vi "Correct U16 Image Array.vi"(8 "Error In":errorcluster, 11 "Image Pixels (U16)":u16[][](array[numeric])) -> (0 "Error Out":errorcluster, 3 "Corrected Image Pixels (U16)":u16[][](array[numeric]))   [LabVIEW 2021, in "Image.lvlib"]
doc: "Subtract 32768 from a U16 array if that it its minimum, as is the case for image data read from TIFF files"
uses:
  Image/Image.lvlib
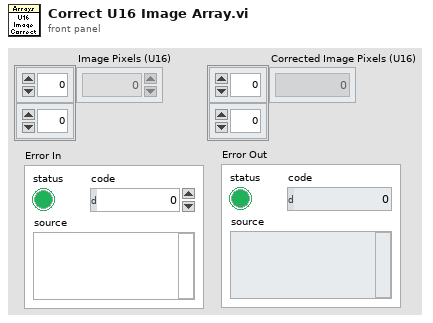
[diagram p1: front panel]
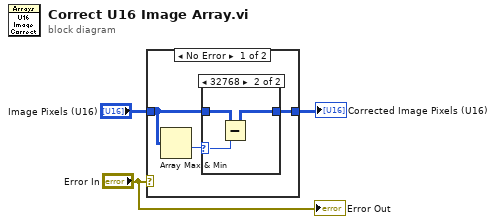
[diagram p0: block diagram]
diagram:
  n1 = case shown="No Error" "Error In" {
    tunnel: "Image Pixels (U16)" -> [w5 w11]
    tunnel: [w4 w11] -> w2
    frame No Error {
      n2 = Array Max & Min(array=w5) -> (min value=w6:u16)  [unwired: 3 out]
      n3 = case shown="32768" w6 {
        selector: w6 -> [_ w9]
        tunnel: w5 -> [w7 w10]
        tunnel: [w7 w8] -> w4
        frame 0, Default {
        }
        frame 32768 {
          n4 = Subtract(x=w10, y=w9) -> (x-y=w8:u16[][])
        }
      }
    }
    frame Error {
    }
  }
  "Corrected Image Pixels (U16)" <- w2
  "Error Out" <- "Error In"
